vi "Configure.vi"(8 "error in (no error)":errorcluster, 9 "Default Path":path, 10 "Interactive?":bool, 11 "Report In":refnum<class "Report.lvclass">) -> (0 "error out":errorcluster, 3 "Report Out":refnum<class "Report.lvclass">)   [LabVIEW 2020, in "Report Generation.lvlib" / "Report.lvclass"]
uses:
  Report.lvclass
  Report.lvclass/Report.ctl
  Report Generator/Report Generator.lvclass
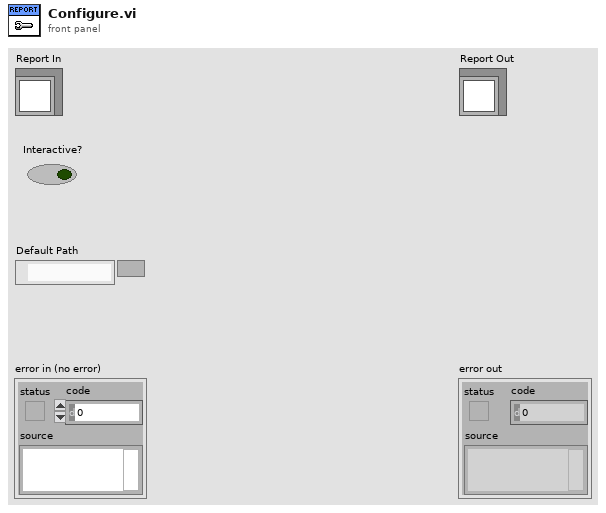
[diagram p1: front panel]
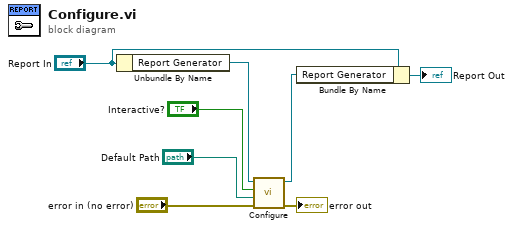
[diagram p0: block diagram]
diagram:
  n1 = Unbundle By Name("Report In") -> ("Report Generator"=w7:refnum<class "Report Generator.lvclass">)
  n2 = call "Configure.vi"("error in (no error)"="error in (no error)", "Default Path"="Default Path", "Interactive?"="Interactive?", "Report Generator in"=w7) -> ("error out"=→"error out":errorcluster, "Report Generator out"=w1:refnum<class "Report Generator.lvclass">)  [unwired: 6 in]
  n3 = Bundle By Name(cluster="Report In", "Report Generator"=w1) -> (→"Report Out":refnum<class "Report.lvclass">)
